vi "PH_VacuumControl.constructor.vi"(0 "name":string, 2 "data in":string, 5 "error in(no error)":errorcluster) -> (14 "i ref out":refnum<vi>, 16 "data out":string, 19 "error out":errorcluster)   [LabVIEW 2014, in "PH_VacuumControl.lvlib"]
doc: "This class reads out an AGCxxx vacuum controller. Also the unit can be set. \n\nThis class is part of the PHELIX device layer.\n\nauthor: Stefan Götte, GSI\n\nLicense Agreement for this software:\n\nCopyright (C)\nGesellschaft für Schwerionenforschung, GSI\nPlanckstr. 1\n64291 Darmstadt\nGermany\n\nContact: D.Beck@gsi.de \n\nThis program is free software; you can redistribute it and/or modify it under the terms of the \nGNU General Public License as published by the Free Software Foundation; either version 2 of \nthe license, or (at your option) any later version.\n\nThis program is distributed in the hope that it will be useful, but WITHOUT ANY WARRANTY; \nwithout even the implied warranty of MERCHANTABILITY or FITNESS FOR A PARTICULAR PURPOSE. See the GNU General License for more details (http://www.gnu.org).\n\nGesellschaft für Schwerionenforschung, GSI\nPlanckstr. 1, 64291 Darmstadt, Germany\nFor all questions and ideas contact: M.Richter@gsi.de, H.Brand@gsi.de or D.Beck@gsi.de.\nLast update: 16-JUN-2004"
uses:
  PH_VacuumControl.lvlib
  PH_Basics/PH_StatusHandler/PH_StatusHandler.Status.ctl
  PH_Basics/PH_PSDBWriter/PH_PSDBWriter.lvlib
  PH_Basics/PH_Class/PH_Class.lvlib
  PH_Basics/PH_StatusHandler/PH_StatusHandler.lvlib
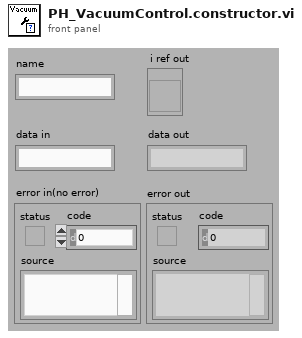
[diagram p1: front panel]
types:
  T1 = enum16{"SetAttribute", "GetAttribute", "CreateAttribute", "DestroyAttribute", "DestroyAllAtributes"}
  T2 = typedef "PH_VacuumControl.lvlib/PH_VacuumControl.i attribute.ctl" = cluster{"GUI Refs":cluster{"Exit":refnum<vi>, "Set Unit":refnum<vi>, "Device found":refnum<vi>, "Busy":refnum<vi>, "State":refnum<vi>, "Delete":refnum<vi>, "Channels":refnum<vi>, "Channel Name":refnum<vi>, "Trend":refnum<vi>, "Logarithmic":refnum<vi>, "Limit reached":refnum<vi>, "Channel Name 1 MT":refnum<vi>, "Channel Name 2 MT":refnum<vi>, "Trend MT":refnum<vi>, "Logarithmic MT":refnum<vi>, "Limit reached MT":refnum<vi>}, "Device found":bool, "Busy":bool, "Selected Unit":i32, "Channels [mbar]":T3, "Channel Names":cluster{"Channel 1":string, "Channel 2":string, "Channel 3":string, "Channel 4":string, "Channel 5":string, "Channel 6":string}, "Status":T4, "AGCxxx VISA Cluster":T5, "Instr Firmware Revision":string, "Service IDs Pressure":cluster{"Channel 1":i32, "Channel 2":i32, "Channel 3":i32, "Channel 4":i32, "Channel 5":i32, "Channel 6":i32}, "Service IDs Limits":cluster{"Channel 1":i32, "Channel 2":i32, "Channel 3":i32, "Channel 4":i32, "Channel 5":i32, "Channel 6":i32}, "Trend":cluster{"Start Point":timestamp, "Pressures [mbar] Channel 1":dbl[], "Pressures [mbar] Channel 2":dbl[], "Pressures [mbar] Channel 3":dbl[], "Pressures [mbar] Channel 4":dbl[], "Pressures [mbar] Channel 5":dbl[], "Pressures [mbar] Channel 6":dbl[], "Timebase [s]":i32[], "Trend Channel":u16, "Start Fit":dbl, "Trend Channel 1 MT":u16, "Trend Channel 2 MT":u16, "Start or continue Fit MT":dbl, "Continue or start Fit MT":dbl, "Datasets strored":i32, "Dataarray Size":i32}, "Running":bool}
  T3 = typedef "PH_VacuumControl.lvlib/PH_VacuumControl.Channels.ctl" = cluster{"Channel 1":dbl, "Channel 2":dbl, "Channel 3":dbl, "Channel 4":dbl, "Channel 5":dbl, "Channel 6":dbl, "Name Channel 1":string, "Name Channel 2":string, "Name Channel 3":string, "Name Channel 4":string, "Name Channel 5":string, "Name Channel 6":string, "Upper Limit":dbl, "Upper Limit 2":dbl, "Upper Limit 3":dbl, "Upper Limit 4":dbl, "Upper Limit 5":dbl, "Upper Limit 6":dbl}
  T4 = typedef "PH_StatusHandler.lvlib/PH_StatusHandler.Status.ctl" = i16
  T5 = typedef "AGCxxx - Driver.lvlib/AGCxxx VISA Control.ctl" = cluster{"VISA resource name":refnum<visa-resource-name>, "VISA Timeout Value (1000 ms)":u32, "Lock Timeout (1000 ms)":u32, "MAX Channel (6)":i32}
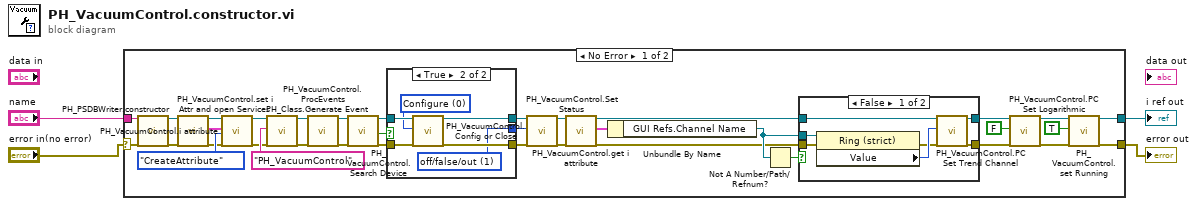
[diagram p0: block diagram]
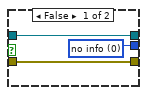
[diagram p3: hidden frame]
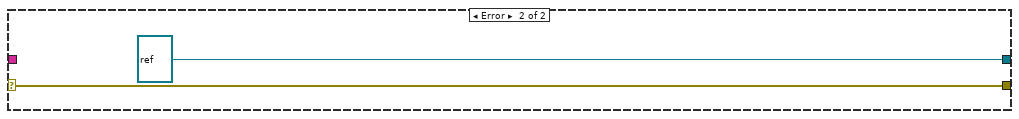
[diagram p4: hidden frame]
diagram:
  n1 = case shown="No Error" "error in(no error)" {
    selector: "error in(no error)" -> [w11 w60]
    tunnel: "name" -> [w34 _]
    tunnel: [w8 refnum<vi> refnum ("i ref out")] -> w3
    tunnel: [w10 w60] -> w2
    frame No Error {
      n2 = call "PH_PSDBWriter.constructor.vi"("name"=w34, "error in"=w11) -> ("i ref out"=w6:refnum<vi>, "error out"=w5:errorcluster)  [unwired: 15 in, 1 out]
      n3 = call "PH_VacuumControl.set i Attr and open Services.vi"("i ref in"=w6, "error in (no error)"=w5) -> ("i ref out"=w16:refnum<vi>, "i Attributes"=w15:T2, "error out"=w12:errorcluster)  [unwired: 15 in]
      n4 = call "PH_VacuumControl.i attribute.vi"("VI Refnum"=w16, "CLASS.i attribute"=w15, "Action"=T1."CreateAttribute", "error in (no error)"=w12) -> ("VI Refnum out"=w14:refnum<vi>, "error out"=w13:errorcluster)  [unwired: 13 in, 1 out]
      n5 = call "PH_Class.Generate Event.vi"("i ref in"=w14, "Class"="PH_VacuumControl", "error in (no error)"=w13) -> ("i ref out"=w20:refnum<vi>, "error out"=w19:errorcluster)  [unwired: 15 in]
      n6 = call "PH_VacuumControl.ProcEvents.vi"("i ref in"=w20, "error in"=w19) -> ("i ref out"=w22:refnum<vi>, "error out"=w21:errorcluster)  [unwired: 16 in]
      n7 = call "PH_VacuumControl.Search Device.vi"("i ref in"=w22, "error in (no error)"=w21) -> ("i ref out"=w40:refnum<vi>, "Device found"=w36:bool, "error out"=w38:errorcluster)  [unwired: 15 in]
      n8 = case shown="True" w36 {
        tunnel: w40 -> [w50 w58]
        tunnel: [w50 w57] -> w39
        tunnel: w38 -> [w51 w56]
        tunnel: [w51 w55] -> w37
        tunnel: [w52 w54] -> w35
        frame False {
          w52 = T4 0 items=["no info", "off/false/out", "on/true/in", "Failure", "Alarm", "Status 1", "Status 2", "Status 3"] ("State")
        }
        frame True {
          w53 = u16 0 items=["Configure", "Close"] ("Action")
          w54 = T4 1 items=["no info", "off/false/out", "on/true/in", "Failure", "Alarm", "Status 1", "Status 2", "Status 3"] ("State")
          n9 = call "PH_VacuumControl.Config or Close.vi"("i ref in"=w58, "Action"=w53, "error in (no error)"=w56) -> ("i ref out"=w57:refnum<vi>, "error out"=w55:errorcluster)  [unwired: 15 in]
        }
      }
      n10 = call "PH_VacuumControl.Set Status.vi"("i ref in"=w39, "Status"=w35, "error in (no error)"=w37) -> ("i ref out"=w24:refnum<vi>, "error out"=w23:errorcluster)  [unwired: 15 in]
      n11 = call "PH_VacuumControl.get i attribute.vi"("i ref in"=w24, "error in (no error)"=w23) -> ("i ref out"=w29:refnum<vi>, "i attribute"=w33:T2, "error out"=w30:errorcluster)  [unwired: 15 in]
      n12 = Unbundle By Name(w33) -> ("GUI Refs.Channel Name"=w31:refnum<vi>)
      n13 = Not A Number/Path/Refnum?(number/path/refnum=w31) -> (NaN/Path/Refnum?=w32:bool)
      n14 = case shown="False" w32 {
        tunnel: w30 -> [w47 w48]
        tunnel: w31 -> [w46 _]
        tunnel: w29 -> [w45 w49]
        tunnel: [w44 w49] -> w27
        tunnel: [w41 w48] -> w28
        frame False {
          n15 = property class="Ring (strict)"(reference=w46, error in=w47) -> (error out=w42:errorcluster, "Value"=w43:u16)  [unwired: 1 out]
          n16 = call "PH_VacuumControl.PC Set Trend Channel.vi"("i ref in"=w45, "Trend Channel"=w43, "error IO"=w42) -> ("i ref out"=w44:refnum<vi>, "error out"=w41:errorcluster)  [unwired: 15 in]
        }
        frame True {
        }
      }
      n17 = call "PH_VacuumControl.PC Set Logarithmic.vi"("i ref in"=w27, "Logarithmic"=FALSE, "error IO"=w28) -> ("i ref out"=w9:refnum<vi>, "error out"=w25:errorcluster)  [unwired: 15 in]
      n18 = call "PH_VacuumControl.set Running.vi"("VI in"=w9, "Running"=TRUE, "error in (no error)"=w25) -> ("VI out"=w8:refnum<vi>, "error out"=w10:errorcluster)  [unwired: 15 in]
    }
    frame Error {
    }
  }
  "i ref out" <- w3
  "error out" <- w2
